vi "Basic Toggle.vi"(5 "Input":bool) -> (2 "Output":bool)   [LabVIEW 2014]
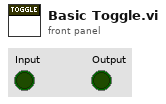
[diagram p1: front panel]
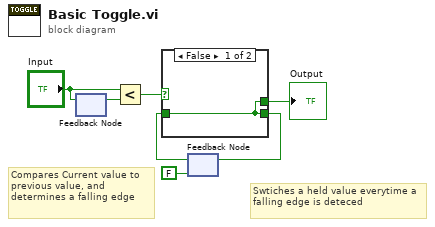
[diagram p0: block diagram]
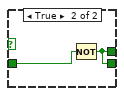
[diagram p2: hidden frame]
diagram:
  # "Swtiches a held value everytime a falling edge is deteced"
  # "Compares Current value to previous value, and determines a falling edge"
  n1 = feedback-in #1("Input") -> ()
  n2 = feedback #1() -> (w6:bool)  [unwired: 1 in]
  n3 = Less?(x="Input", y=w6) -> (x < y?=w7:bool)
  n4 = feedback #2(FALSE) -> (w2:bool)
  n5 = case shown="False" w7 {
    tunnel: [w8 w9] -> w4
    tunnel: w2 -> [w8 w10]
    tunnel: [w8 w9] -> w1
    frame False {
    }
    frame True {
      n6 = Not(x=w10) -> (.not. x?=w9:bool)
    }
  }
  "Output" <- w4
  n7 = feedback-in #2(w1) -> ()
